vi "Button Pressed.vi"(8 "error in (no error)":errorcluster, 10 "Button Text":string, 11 "Grid Screen in":refnum<class "Grid Screen.lvclass">) -> (0 "error out":errorcluster, 3 "Grid Screen out":refnum<class "Grid Screen.lvclass">)   [LabVIEW 2021, in "Grid Screen.lvlib" / "Grid Screen.lvclass"]
uses:
  Grid Screen.lvclass
  C:/Program Files/National Instruments/LabVIEW 2024/vi.lib/ActorFramework/Actor/Actor.lvclass
  <vilib>/ActorFramework/Actor/Actor.lvclass/Actor.ctl
  Grid Screen.lvclass/Grid Screen.ctl
  Controller/Controller Messages/Retrieve Question Msg/Retrieve Question Msg.lvclass/Retrieve Question Msg.ctl
  <vilib>/ActorFramework/Message Enqueuer/Message Enqueuer.lvclass/Message Enqueuer.ctl
  <vilib>/ActorFramework/Message Enqueuer/Enqueue.vi
  Controller/Controller Messages/Retrieve Question Msg/Retrieve Question Msg.lvclass
  C:/Program Files/National Instruments/LabVIEW 2024/vi.lib/ActorFramework/Message/Message.lvclass
  <vilib>/ActorFramework/Message Priority Queue/Priority Enqueue.vi
  <vilib>/ActorFramework/Actor/Actor.lvclass
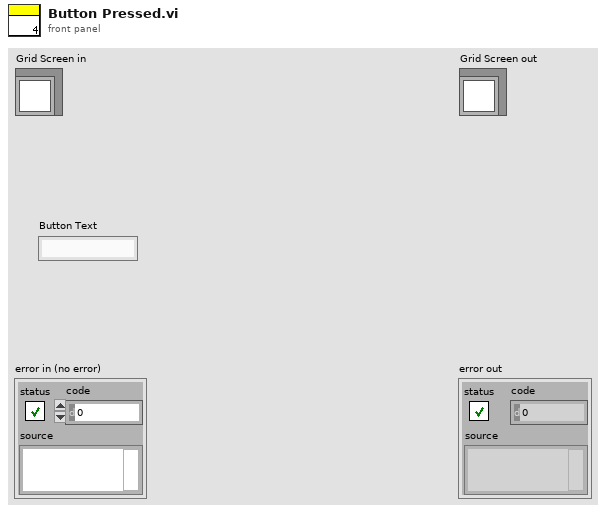
[diagram p1: front panel]
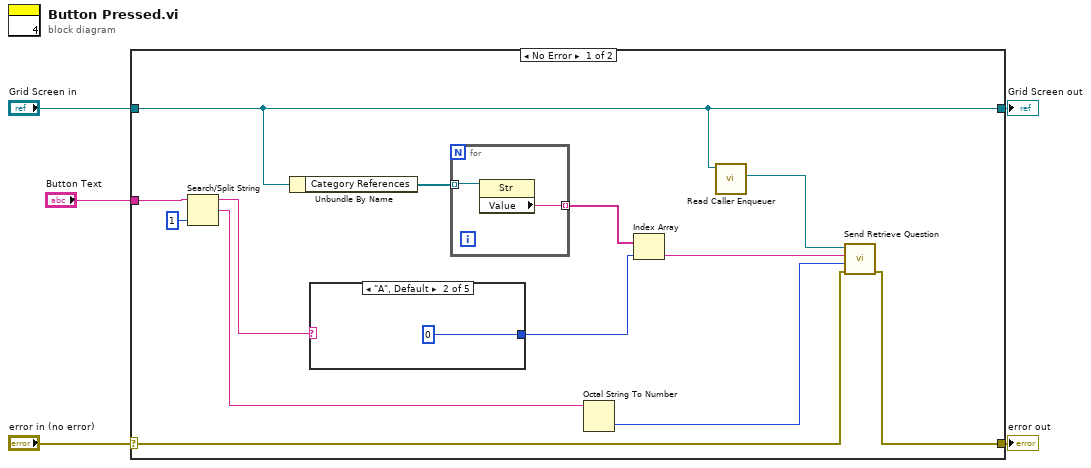
[diagram p0: block diagram]
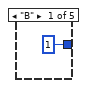
[diagram p2: hidden frame]
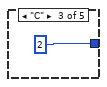
[diagram p3: hidden frame]
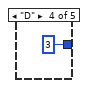
[diagram p4: hidden frame]
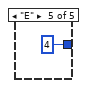
[diagram p5: hidden frame]
diagram:
  n1 = case shown="No Error" "error in (no error)" {
    selector: "error in (no error)" -> [w7 w27]
    tunnel: [w6 w27] -> w4
    tunnel: [w9 w26] -> w2
    tunnel: "Grid Screen in" -> [w9 w26]
    tunnel: "Button Text" -> [w17 _]
    frame No Error {
      n2 = Search/Split String(string=w17, offset (0)=1) -> (substring before match=w14:string, match + rest of string=w12:string)  [unwired: 1 in, 1 out]
      n3 = Unbundle By Name(w9) -> ("Category References"=w16:refnum<vi>[])
      n4 = case shown="\"A\", Default" w14 {
        tunnel: [1 ("index") 0 ("index") 2 ("index") 3 ("index") 4 ("index")] -> w13
        frame "B" {
        }
        frame "A", Default {
        }
        frame "C" {
        }
        frame "D" {
        }
        frame "E" {
        }
      }
      n5 = for {
        tunnel: w16 -> [w25] mode=indexing
        tunnel: [w24] -> w15 mode=indexing
        n6 = property class="Str"(reference=w25) -> ("Value"=w24:string)  [unwired: 1 in, 2 out]
      }
      n7 = Octal String To Number(4:w12) -> (0:w10:u32)  [unwired: 2 in, 1 out]
      n8 = Index Array(array=w15, index=w13) -> (element=w11:string)
      n9 = call <vilib>:"Read Caller Enqueuer.vi"("Actor"=w9) -> ("Caller Enqueuer"=w8:refnum<class "Message Enqueuer.lvclass">)  [unwired: 10 in]
      n10 = call "Send Retrieve Question.vi"("error in (no error)"=w7, "Difficulty"=w10, "Category"=w11, "Message Enqueuer"=w8) -> ("error out"=w6:errorcluster)  [unwired: 6 in, 1 out]
    }
    frame Error {
    }
  }
  "error out" <- w4
  "Grid Screen out" <- w2
